vi "Delete Tools.vi"(10 "Tools":i32[](array[numeric]), 11 "Server Creator Data in":T1) -> (3 "Server Creator Data out":T1)   [LabVIEW 2025, in "Tools.lvlib"]
uses:
  Tools.lvlib
  Server Creator Data.ctl
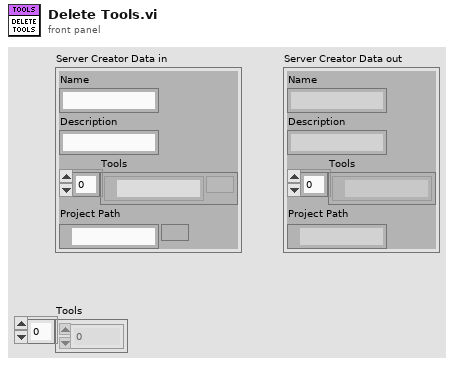
[diagram p1: front panel]
types:
  T1 = typedef "Tools.lvlib/Server Creator Data.ctl" = cluster{"Name":string, "Description":string, "Tools":path[], "Project Path":path}
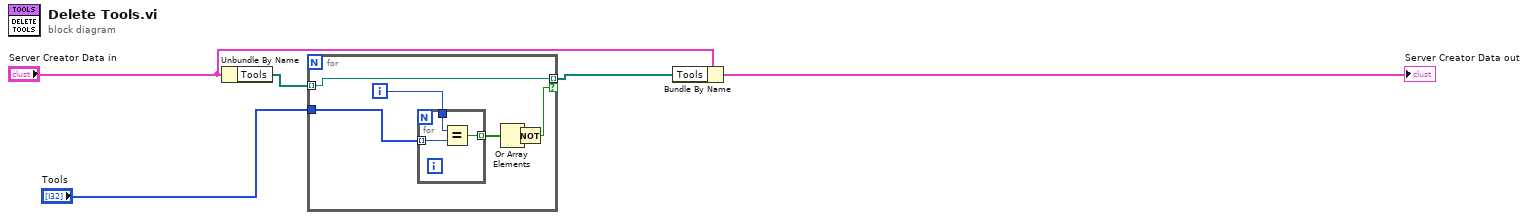
[diagram p0: block diagram]
diagram:
  n1 = Unbundle By Name("Server Creator Data in") -> ("Tools"=w3:path[])
  n2 = for {
    tunnel: w3 -> [w9] mode=indexing
    tunnel: "Tools" -> [w10]
    tunnel: [w9] -> w5 mode=indexing if=w6
    i -> [w11]
    n3 = for {
      tunnel: w11 -> [w14]
      tunnel: w10 -> [w13] mode=indexing
      tunnel: [w12] -> w8 mode=indexing
      n4 = Equal?(x=w14, y=w13) -> (x = y?=w12:bool)
    }
    n5 = Or Array Elements(Boolean array=w8) -> (logical OR=w7:bool)
    n6 = Not(x=w7) -> (.not. x?=w6:bool)
  }
  n7 = Bundle By Name(cluster="Server Creator Data in", "Tools"=w5) -> (→"Server Creator Data out":T1)
